vi "Write_real.vi"() -> ()   [LabVIEW 2023]
uses:
  <vilib>/OPCUA/controls/NodeId.ctl
  <vilib>/OPCUA/controls/Write Status.ctl
  <vilib>/OPCUA/client/Multiple Write Double.vi
  <vilib>/OPCUA/NI OPC UA Client.lvlib
panel:
  in  "Sensor type":string(combo)="TC01"
  in  "Stop Button":bool
  in  "Item Path":string="ns=2;s=Tag1"
  out "Temperature from DAQ":dbl
  in  "Server Endpoint URL":string="opc.tcp://beist:62640/IntegrationObjects/ServerSimulator"
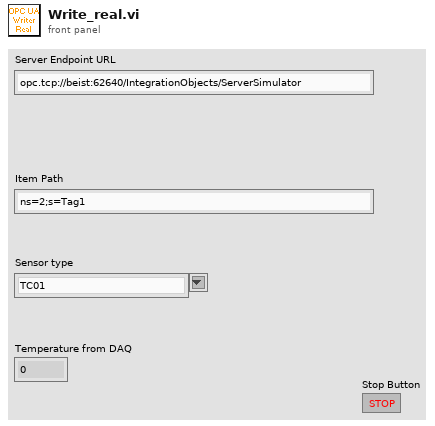
[diagram p1: front panel]
types:
  T1 = cluster{"message mode":enum16{"None", "Sign", "Sign and Encrypt"}, "security":enum16{"Basic256", "Basic128Rsa15"}}
  T2 = typedef "OPC UA Client Refnum.ctl" = refnum<k21>
  T3 = typedef "NodeId.ctl" = string
  T4 = typedef "Write Status.ctl" = u32
  T5 = cluster{"node ID":T3, "value":dbl, "timestamp (current time)":timestamp, "node status":T4}
  T6 = cluster{"node ID":T3, "value":dbl, "timestamp (current time)":timestamp, "node status":T4}[]
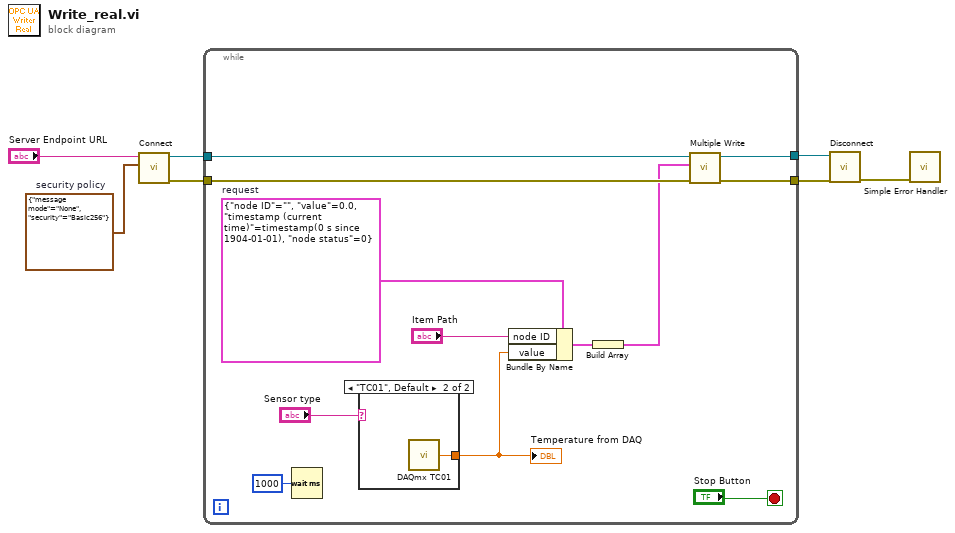
[diagram p0: block diagram]
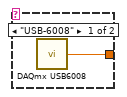
[diagram p2: hidden frame]
diagram:
  w7 = T1 {"message mode"=enum."None", "security"=enum."Basic256"}  # security policy
  n1 = call <vilib>:"Connect.vi"("security policy"=w7, "server endpoint URL"="Server Endpoint URL") -> ("error out"=w4:errorcluster, "OPC UA client refnum out"=w6:T2)  [unwired: 7 in, 1 out]
  n2 = while {
    tunnel: w6 -> [w17]
    tunnel: [w16] -> w5
    tunnel: w4 -> [w15]
    tunnel: [w14] -> w3
    stop <- "Stop Button" stop-if-true
    w11 = T5 {"node ID"="", "value"=0.0, "timestamp (current time)"=timestamp(0 s since 1904-01-01), "node status"=0}  # request
    n3 = Wait (ms)(milliseconds to wait=u32 1000) -> ()  [unwired: 1 out]
    n4 = case shown="\"TC01\", Default" "Sensor type" {
      tunnel: [w20 w21] -> w9
      frame "USB-6008" {
        n5 = call "DAQmx USB6008.vi"() -> ("Temperature data"=w20:dbl)  [unwired: 1 in]
      }
      frame "TC01", Default {
        n6 = call "DAQmx TC01.vi"() -> ("Temperature data"=w21:dbl)  [unwired: 1 in]
      }
    }
    "Temperature from DAQ" <- w9
    n7 = Bundle By Name "Bundle By Name"(cluster=w11, "node ID"="Item Path", "value"=w9) -> (w12:T5)
    n8 = Build Array "Build Array"(w12) -> (w10:T6)
    n9 = call-poly <vilib>:"Multiple Write.vi"("error in (no error)"=w15, "requests"=w10, "OPC UA client refnum in"=w17) -> ("error out"=w14:errorcluster, "OPC UA client refnum out"=w16:T2)  [unwired: 5 in, 2 out]
  }
  n10 = call <vilib>:"Disconnect.vi"("error in (no error)"=w3, "OPC UA client refnum in"=w5) -> ("error out"=w2:errorcluster)  [unwired: 9 in]
  n11 = call <vilib>:"Simple Error Handler.vi"("error in (no error)"=w2) -> ()  [unwired: 4 in, 5 out]
